vi "Get Virt Instrs.vi"(11 "MSS in":refnum<class "MSS.lvclass">) -> (2 "Virt Instrs":T1(c390), 3 "MSS out":refnum<class "MSS.lvclass">)   [LabVIEW 2024, in "HAL.lvlib" / "MSS.lvclass"]
uses:
  MSS.lvclass
  Virtual Instruments/Virtual Instrument/Virtual Instrument.lvclass
  MSS.lvclass/MSS.ctl
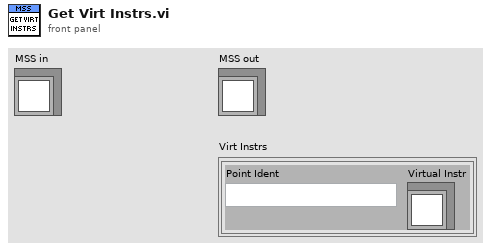
[diagram p1: front panel]
types:
  T1 = map{string, refnum<class "Virtual Instrument.lvclass">}
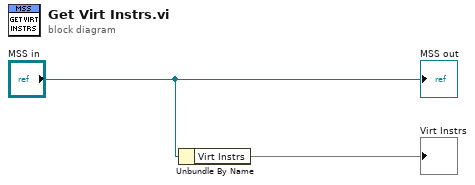
[diagram p0: block diagram]
diagram:
  n1 = Unbundle By Name("MSS in") -> ("Virt Instrs"=→"Virt Instrs":T1)
  "MSS out" <- "MSS in"
